vi "PPMS temperature.vi"(2 "error in (no error)":errorcluster, 3 "Transmit Mode (0)":T1(ring), 4 "GPIB address":string="15") -> (0 "error out":errorcluster, 1 "Temperature (K)":dbl format="%.3f")   [LabVIEW 2017]
doc: "This returns the temperature of the sample chamber according to the user configured thermometer in kelvin."
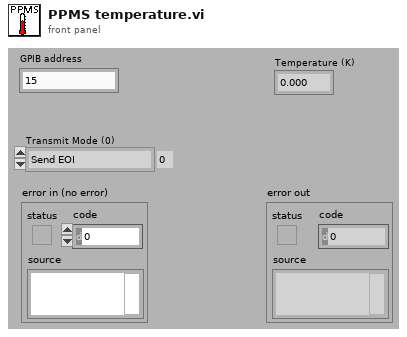
[diagram p1: front panel]
types:
  T1 = enum16{"Send EOI", "append CR w/ EOI", "append LF w/ EOI", "append CR LF w/ EOI", "append CR w/o EOI", "append LF w/o EOI", "append CR LF w/o EOI", "do not send EOI"}
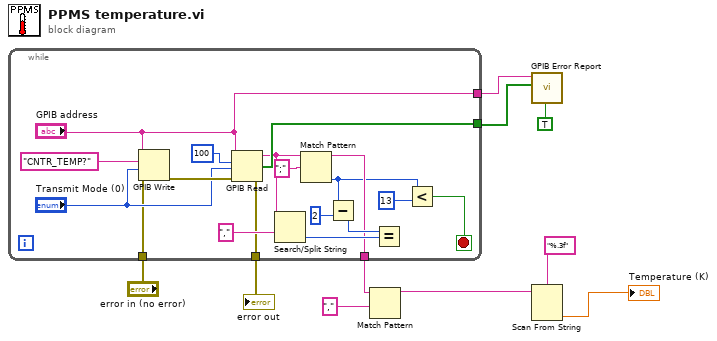
[diagram p0: block diagram]
diagram:
  n1 = while {
    tunnel: ["GPIB address"] -> w9
    tunnel: [w23] -> w8
    tunnel: [w15] -> w3
    tunnel: [w12] -> w2
    tunnel: "error in (no error)" -> [w11]
    stop <- w24 stop-if-true
    n2 = GPIB Write(0:"GPIB address", 1:"CNTR_TEMP?", 2:"Transmit Mode (0)", 3:w11) -> (6:w27:errorcluster)  [unwired: 1 in, 1 out]
    n3 = GPIB Read(0:"GPIB address", 1:100, 2:"Transmit Mode (0)", 3:w27) -> (5:w14:string, 6:w23:bool[], 7:w12:errorcluster)  [unwired: 1 in]
    n4 = Search/Split String(string=w14, search string/char (-)=",") -> (offset of match=w18:i32)  [unwired: 1 in, 2 out]
    n5 = Match Pattern(string=w14, regular expression=";") -> (before substring=w15:string, offset past match=w13:i32)  [unwired: 1 in, 2 out]
    n6 = Subtract(x=w13, y=2) -> (x-y=w17:i32)
    n7 = Equal?(x=w17, y=w18) -> ()  [unwired: 1 out]
    n8 = Less?(x=w13, y=13) -> (x < y?=w24:bool)
  }
  "error out" <- w2
  n9 = Match Pattern(string=w3, regular expression=",") -> (before substring=w4:string)  [unwired: 1 in, 3 out]
  n10 = call "GPIB Error Report.vi"("Dialog?(F)"=TRUE, "Status"=w8, "Address String"=w9) -> ()  [unwired: 1 in, 2 out]
  n11 = Scan From String(format string="%.3f", input string=w4) -> (output 1=→"Temperature (K)":dbl)  [unwired: 3 in, 3 out]
